vi "Send.vi"(8 "error in (no error)":errorcluster, 10 "Data Notification":refnum<class "Data.lvclass">, 11 "Notifier in":refnum<class "Notifier.lvclass">) -> (0 "error out":errorcluster, 3 "Notifier out":refnum<class "Notifier.lvclass">)   [LabVIEW 2020, in "Data.lvlib" / "Notifier.lvclass"]
doc: "Send a notification."
uses:
  Notifier.lvclass
  Data.lvclass
  Notifier.lvclass/Notifier.ctl
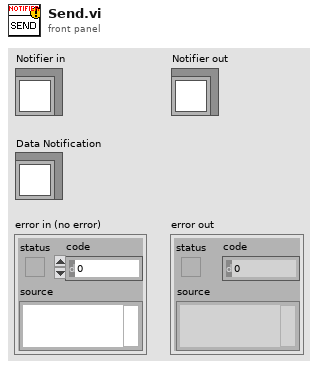
[diagram p1: front panel]
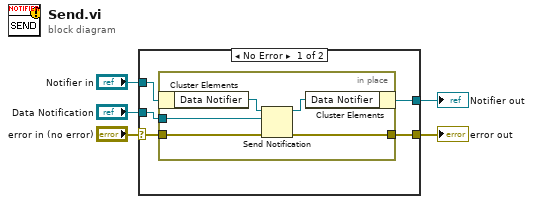
[diagram p0: block diagram]
diagram:
  n1 = case shown="No Error" "error in (no error)" {
    selector: "error in (no error)" -> [w8 w17]
    tunnel: [w7 w17] -> w4
    tunnel: [w9 w16] -> w2
    tunnel: "Notifier in" -> [w10 w16]
    tunnel: "Data Notification" -> [w6 _]
    frame No Error {
      n2 = in-place {
        in-place-border: w8 -> [w13]
        in-place-border: [w12] -> w7
        in-place-border: w6 -> [w11]
        n3 = in-place-cluster #1(w10) -> ("Data Notifier"=w15:refnum<notifier>)
        n4 = Send Notification(notification=w11, notifier=w15, error in (no error)=w13) -> (notifier out=w14:refnum<notifier>, error out=w12:errorcluster)
        n5 = in-place-cluster #1("Data Notifier"=w14) -> (w9:refnum<class "Notifier.lvclass">)
      }
    }
    frame Error {
    }
  }
  "error out" <- w4
  "Notifier out" <- w2
